vi "DCMotor VelocityChangeEvent Example.vi"() -> ()   [LabVIEW 2012, in "Phidget DC Motor.lvlib"]
uses:
  <instrlib>/Phidgets/Phidget DC Motor/Phidget DC Motor.lvlib
  <instrlib>/Phidgets/Phidget DC Motor/Public/DCMotorStart.vi
  <instrlib>/Phidgets/Phidget DC Motor/Public/DCMotorClose.vi
  <instrlib>/Phidgets/Phidget Common/Phidget Common.lvlib
panel:
  out "Velocity Return":dbl caption="Duty Cycle Return"
  in  "Acceleration":dbl=1.0
  in  "Velocity":dbl=1.0 caption="Duty Cycle"
  in  "stop":bool
  out "Serial Number Return":i32
  in  "Device Info":T1={"Serial Number"=-1, "Channel"=0, "Port"=0}
  out "error out":errorcluster
  # "Be sure to use this stop button to stop the program.\nIf you use the \"Abort Execution\" button, you will\nneed to use PhidgetResetLibrary.vi or restart Labview \nin order for any Phidgets to work."
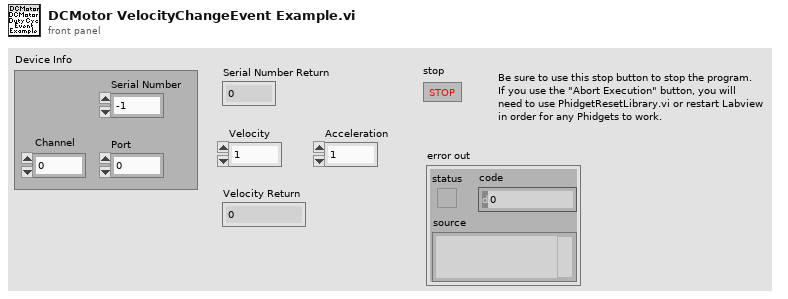
[diagram p1: front panel]
types:
  T1 = cluster{"Serial Number":i32, "Channel":i32, "Port":i32}
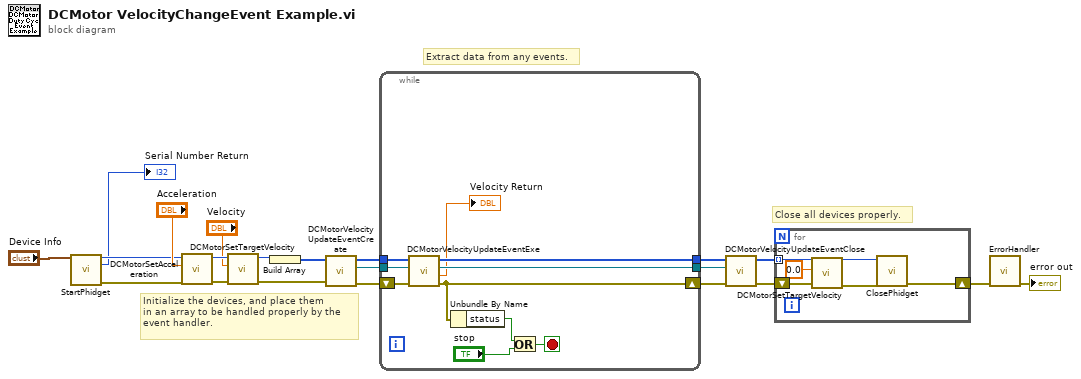
[diagram p0: block diagram]
diagram:
  # "Close all devices properly."
  # "Extract data from any events."
  # "Initialize the devices, and place them\nin an array to be handled properly by the\nevent handler."
  n1 = call-poly <instrlib>:"StartPhidget.vi"("Device Info"="Device Info") -> ("Phidget ID"=w3:u64, "Serial Number Return"=→"Serial Number Return":i32, "error out"=w2:errorcluster)  [unwired: 11 in, 1 out]
  n2 = call <instrlib>:"DCMotorSetAcceleration.vi"("error in (no error)"=w2, "Acceleration"="Acceleration", "Device In"=w3) -> ("error out"=w9:errorcluster, "Device Out"=w8:u64)  [unwired: 6 in]
  n3 = call <instrlib>:"DCMotorSetTargetVelocity.vi"("error in (no error)"=w9, "Velocity"="Velocity", "Device In"=w8) -> ("error out"=w6:errorcluster, "Device Out"=w7:u64)  [unwired: 6 in]
  n4 = Build Array(w7) -> (w21:u64[])
  n5 = call <instrlib>:"DCMotorVelocityUpdateEventCreate.vi"("error in (no error)"=w6, "Devices In"=w21) -> ("error out"=w14:errorcluster, "Event Registration Refnum"=w19:refnum<event-registration>, "Devices Out"=w20:u64[])  [unwired: 7 in]
  n6 = while {
    tunnel: w20 -> [w31]
    tunnel: w19 -> [w28]
    tunnel: [w23] -> w16
    shift-right: [w24] -> w15
    shift-left: w14 -> [w30]
    tunnel: [w29] -> w10
    stop <- w27 stop-if-true
    n7 = call <instrlib>:"DCMotorVelocityUpdateEventExe.vi"("error in (no error)"=w30, "Event Registration Refnum In"=w28, "Devices In"=w31) -> ("error out"=w24:errorcluster, "Velocity"=→"Velocity Return":dbl, "Event Registration Refnum Out"=w23:refnum<event-registration>, "Devices Out"=w29:u64[])  [unwired: 2 in, 3 out]
    n8 = Unbundle By Name(w24) -> ("status"=w25:bool)
    n9 = Or(x=w25, y="stop") -> (x .or. y?=w27:bool)
  }
  n10 = call <instrlib>:"DCMotorVelocityUpdateEventClose.vi"("error in (no error)"=w15, "Event Registration Refnum In"=w16, "Devices In"=w10) -> ("error out"=w12:errorcluster, "Devices Out"=w11:u64[])  [unwired: 7 in]
  n11 = for {
    tunnel: w11 -> [w35] mode=indexing
    shift-right: [w37] -> w18
    shift-left: w12 -> [w36]
    n12 = call <instrlib>:"DCMotorSetTargetVelocity.vi"("error in (no error)"=w36, "Velocity"=0.0 ("Duty Cycle"), "Device In"=w35) -> ("error out"=w33:errorcluster, "Device Out"=w34:u64)  [unwired: 6 in]
    n13 = call-poly <instrlib>:"ClosePhidget.vi"("error in"=w33, "Device In"=w34) -> ("error out"=w37:errorcluster)  [unwired: 9 in]
  }
  n14 = call <instrlib>:"ErrorHandler.vi"("error in"=w18) -> ("error out"=→"error out":errorcluster)  [unwired: 9 in, 1 out]
